vi "_Measure Transfer Function+optimal.vi"() -> ()   [LabVIEW 2014]
uses:
  <vilib>/Analysis/1siggen.llb/Ramp Pattern by Samples.vi
  <vilib>/Analysis/NI_AALBase.lvlib
panel:
  out "Progress":dbl(slide) scale=0.0..1.0
  out "Device ID":string
  in  "?":cluster{"Channel A":u8, "Channel B":u8}={"Channel A"=0, "Channel B"=4} {"Channel A" max=3; "Channel B" min=4 max=7}
  in  "?":T1={"Sweep start [Hz]"=40.0, "Sweep end [Hz]"=20000.0, "Sweep points"=10, "Periods"=1} {"Sweep start [Hz]" min=40.0 max=40000.0; "Sweep end [Hz]" min=40.0 max=40000.0; "Sweep points" min=1 max=100; "Periods" min=1 max=8}
  out "Phase [°]":dbl
  out "Magnitude [dB]":dbl
  out "Number of samples":dbl
  out "Real fs [Hz]":dbl
  out "Measured Signals":waveform(dbl)[](graph)
  out "Phase response":cluster{dbl[], dbl[]}(graph)
  out "Magnitude response":cluster{dbl[], dbl[]}(graph)
  out "VISA Refnum out":refnum<visa-resource-name>
  out "error out":errorcluster
  in  "VISA Refnum in":refnum<visa-resource-name>="COM4"
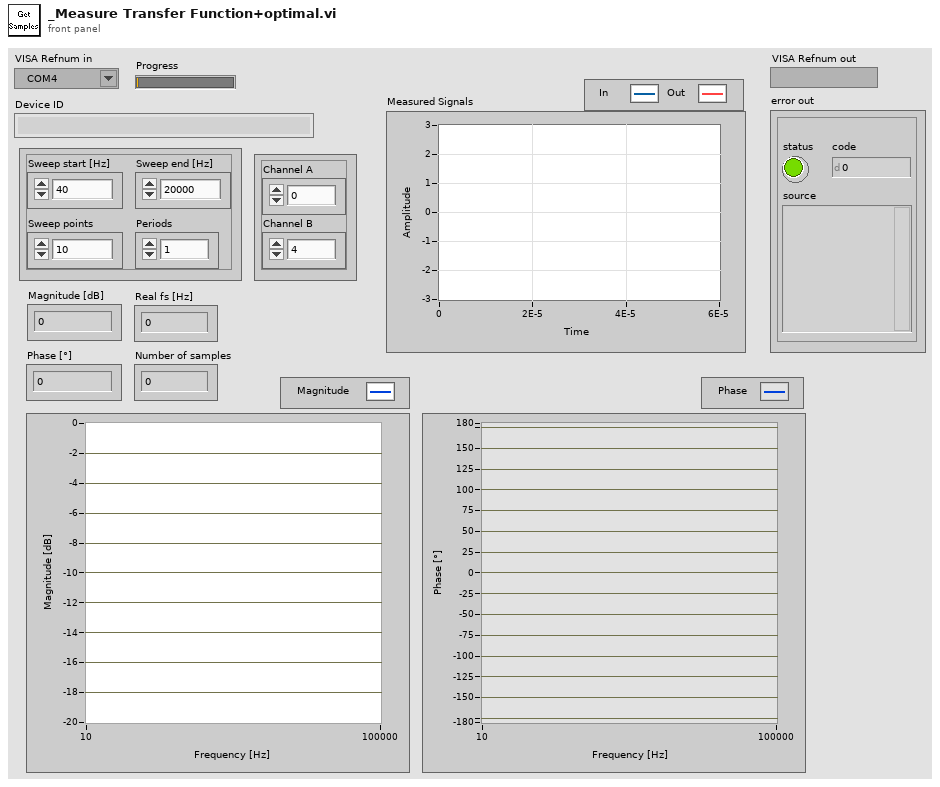
[diagram p1: front panel]
types:
  T1 = cluster{"Sweep start [Hz]":dbl, "Sweep end [Hz]":dbl, "Sweep points":i32, "Periods":u8}
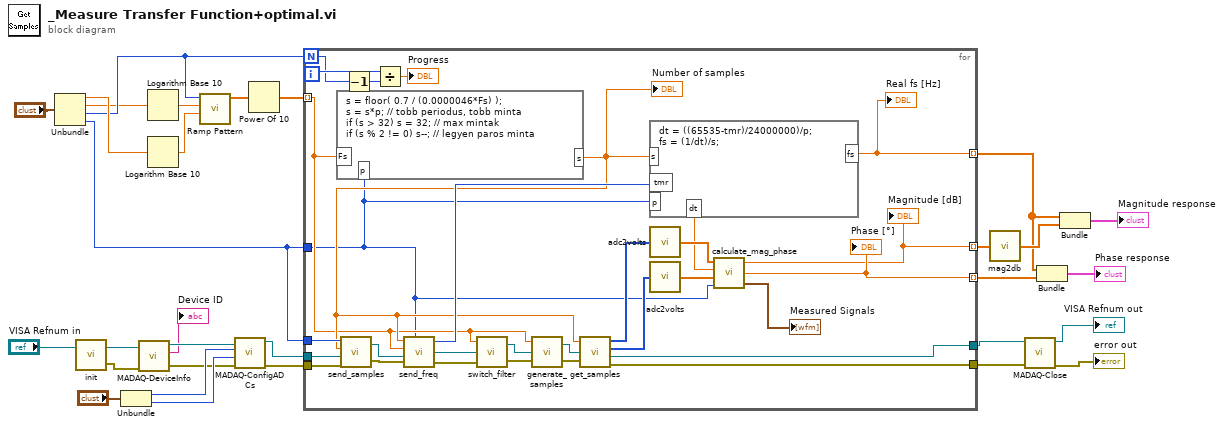
[diagram p0: block diagram]
diagram:
  n1 = Unbundle("?") -> ("Sweep start [Hz]"=w16:dbl, "Sweep end [Hz]"=w14:dbl, "Sweep points"=w15:i32, "Periods"=w13:u8)
  n2 = call "init.vi"("VISA Refnum in"="VISA Refnum in") -> ("error out"=w8:errorcluster, "VISA Refnum out"=w9:refnum<visa-resource-name>)  [unwired: 1 in]
  n3 = Unbundle("?") -> ("Channel A"=w11:u8, "Channel B"=w10:u8)
  n4 = call "MADAQ-DeviceInfo.vi"("error in (no error)"=w8, "VISA resource name"=w9) -> ("error out"=w6:errorcluster, "Device ID"=→"Device ID":string, "VISA resource name out"=w7:refnum<visa-resource-name>)  [unwired: 3 in]
  n5 = Logarithm Base 10(1:w14) -> (0:w29:dbl)
  n6 = Logarithm Base 10(1:w16) -> (0:w28:dbl)
  n7 = call-poly <vilib>:"Ramp Pattern.vi"("start"=w28, "end"=w29, "samples"=w15) -> ("Ramp Pattern"=w30:dbl[])  [unwired: 7 in, 1 out]
  n8 = call "MADAQ-ConfigADCs.vi"("error in (no error)"=w6, "Channel B"=w10, "Channel A"=w11, "VISA resource name"=w7) -> ("error out"=w20:errorcluster, "VISA resource name out"=w21:refnum<visa-resource-name>)  [unwired: 2 in]
  n9 = Power Of 10(x=w30) -> (10^x=w27:dbl[])
  n10 = for {
    N: w15 -> [w32]
    tunnel: w27 -> [w40] mode=indexing
    tunnel: [w55] -> w26
    tunnel: [w54] -> w25
    tunnel: [w49] -> w22 mode=indexing
    tunnel: w13 -> [w46]
    tunnel: w13 -> [w39]
    tunnel: w21 -> [w38]
    tunnel: w20 -> [w37]
    tunnel: [w36] -> w4 mode=indexing
    tunnel: [w35] -> w3 mode=indexing
    i -> [w33]
    n11 = formula code="s = floor( 0.7 / (0.0000046*Fs) );\ns = s*p; // tobb periodus, tobb minta\nif (s > 32) s = 32; // max mintak\nif (s % 2 != 0) s--; // legyen paros minta"("Fs"=w40, "p"=w39) -> ("s"=w45:dbl)
    "Number of samples" <- w45
    n12 = call "send_samples.vi"("error in (no error)"=w37, "VISA Refnum in"=w38, "elemszam"=w45, "periods"=w46) -> ("error out"=w58:errorcluster, "VISA Refnum out"=w59:refnum<visa-resource-name>)
    n13 = Decrement(x=w32) -> (x-1=w31:i32)
    n14 = Divide(x=w33, y=w31) -> (x/y=→"Progress":dbl)
    n15 = call "send_freq.vi"("elemszam"=w45, "signal freq"=w40, "VISA Refnum in"=w59, "error in (no error)"=w58, "periods"=w39) -> ("tmr 2 rld value"=w48:u16, "VISA Refnum out"=w44:refnum<visa-resource-name>, "error out"=w43:errorcluster)
    n16 = call "switch_filter.vi"("error in (no error)"=w43, "VISA Refnum in"=w44, "fs"=w40) -> ("error out"=w42:errorcluster, "VISA Refnum out"=w41:refnum<visa-resource-name>)
    n17 = call "generate_samples.vi"("error in (no error) 2"=w42, "VISA Refnum in 2"=w41, "fs"=w40) -> ("error out"=w56:errorcluster, "VISA Refnum out"=w57:refnum<visa-resource-name>)
    n18 = call "get_samples.vi"("elemszam"=w45, "VISA Refnum in"=w57, "error in (no error)"=w56) -> ("in samples"=w51:u16[], "out samples"=w50:u16[], "VISA Refnum out"=w54:refnum<visa-resource-name>, "error out"=w55:errorcluster)
    n19 = formula code="dt = ((65535-tmr)/24000000)/p;\nfs = (1/dt)/s;"("tmr"=w48, "s"=w45, "p"=w39) -> ("dt"=w47:dbl, "fs"=w35:dbl)
    "Real fs [Hz]" <- w35
    n20 = call "adc2volts.vi"("ADC value"=w51) -> ("Volts"=w53:dbl[])
    n21 = call "adc2volts.vi"("ADC value"=w50) -> ("Volts"=w52:dbl[])
    n22 = call "calculate_mag_phase.vi"("periods"=w39, "OUT samples"=w52, "dt"=w47, "IN samples"=w53) -> ("Measured Signals"=→"Measured Signals":waveform(dbl)[], "Phase"=w49:dbl, "Magnitude"=w36:dbl)
    "Magnitude [dB]" <- w36
    "Phase [°]" <- w49
  }
  n23 = call "mag2db.vi"("Array"=w4) -> ("x*y"=w18:dbl[])
  n24 = call "MADAQ-Close.vi"("error in (no error)"=w26, "VISA resource name"=w25) -> ("error out"=→"error out":errorcluster, "VISA resource name out"=→"VISA Refnum out":refnum<visa-resource-name>)  [unwired: 4 in]
  n25 = Bundle(w3, w22) -> (→"Phase response":cluster{dbl[], dbl[]})  [unwired: 1 in]
  n26 = Bundle(w3, "x*y"=w18) -> (→"Magnitude response":cluster{dbl[], "x*y":dbl[]})  [unwired: 1 in]
